vi "Configure Device.vi"(8 "error in (no error)":errorcluster, 11 "Device in":refnum<class "Device.lvclass">) -> (0 "error out":errorcluster, 3 "Device out":refnum<class "Device.lvclass">)   [LabVIEW 2020, in "HAL.lvlib" / "Device.lvclass"]
doc: "This VI should be overridden to pull configuration values using the base Device class' Lookup Config Value VI and then converting the string value into the data type. Note that all configuration values need to be provided in string format to the base Device class for easy persistence via INI file or other method.\n\nIf there is a problem with a config value's format or a required value is missing, this VI should return an appropriate error so that the Device can track state properly."
uses:
  Device.lvclass
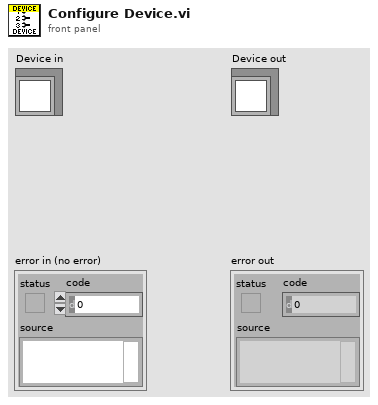
[diagram p1: front panel]
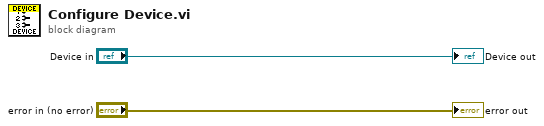
[diagram p0: block diagram]
diagram:
  "error out" <- "error in (no error)"
  "Device out" <- "Device in"
